vi "Stop.vi"(6 "Teller":refnum<class "Teller.lvclass">, 8 "Error in":errorcluster, 9 "Parent Stopped":bool, 10 "Safe Stop":bool=TRUE, 11 "Base Actor in":refnum<class "Base Actor.lvclass">) -> (0 "Error out":errorcluster, 3 "Base Actor out":refnum<class "Base Actor.lvclass">)   [LabVIEW 2025, in "jettl.lvlib" / "Base Actor.lvlib" / "Base Actor.lvclass"]
uses:
  Base Actor.lvclass
  Teller/Teller.lvclass
  Base Actor.lvclass/Base Actor.ctl
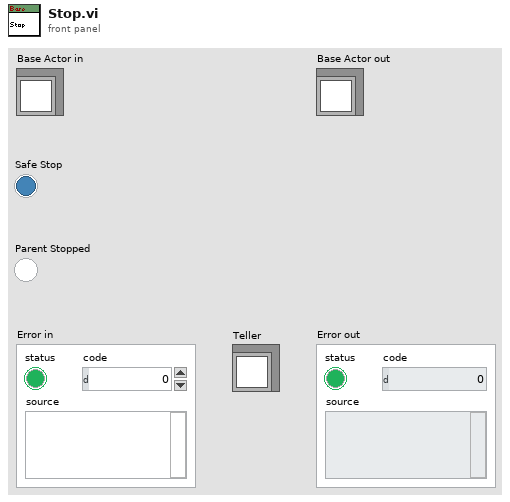
[diagram p1: front panel]
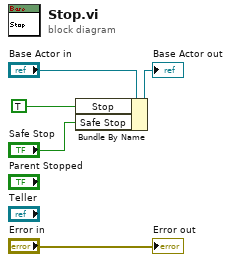
[diagram p0: block diagram]
diagram:
  n1 = Bundle By Name(cluster="Base Actor in", "Stop"=TRUE ("Is Marked For Destroy"), "Safe Stop"="Safe Stop") -> (→"Base Actor out":refnum<class "Base Actor.lvclass">)
  "Error out" <- "Error in"
